vi "LVDimInterface.dic_release_service.vi"(0 "callBackID":i32, 5 "error in (no error)":errorcluster) -> (19 "error out":errorcluster)   [LabVIEW 2014, in "LVDimInterface.lvlib"]
doc: "Unregisters a control from a DIM service."
uses:
  LVDimInterface.lvlib
  bin/libDimWrapper.dll
  bin/libDimWrapper.so
  bin/libDimWrapperSPL.dll
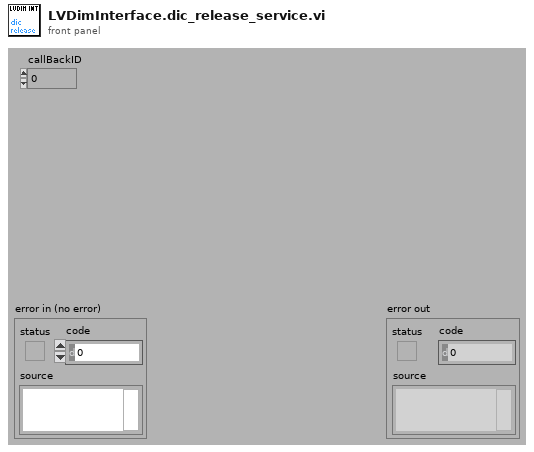
[diagram p1: front panel]
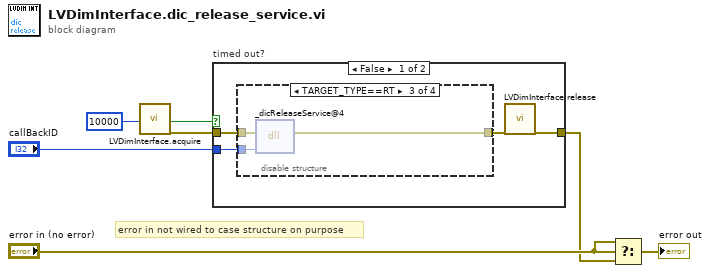
[diagram p0: block diagram]
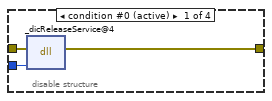
[diagram p2: hidden frame]
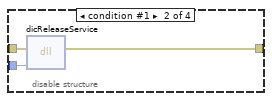
[diagram p3: hidden frame]
diagram:
  # "error in not wired to case structure on purpose"
  n1 = call "LVDimInterface.acquire.vi"("ms timeout (10000)"=10000 ("ms timeout (-1)")) -> ("timed out"=w5:bool, "error out"=w2:errorcluster)  [unwired: 17 in]
  n2 = case "timed out?" shown="False" w5 {
    tunnel: "callBackID" -> [w11 _]
    tunnel: w2 -> [w10 w22]
    tunnel: [w8 w22] -> w1
    frame False {
      n3 = disable-structure "Conditional Disable Structure" shown="TARGET_TYPE==RT" {
        disable-tunnel: w11 -> [w14 w17 w20 _]
        disable-tunnel: w10 -> [w13 w16 w19 w21]
        disable-tunnel: [w12 w15 w18 w21] -> w9
        frame condition #0 (active) {
          n4 = dll-call lib="D:/Git/CS-framework/CSlibraries-extern/DimLVEvent/bin/libDimWrapper.dll" fn="_dicReleaseService@4" label="dic_release_service"(error in=w13, "callBackID"=w14) -> (error out=w12:errorcluster)  [unwired: 4 in, 1 out]
        }
        frame condition #1 {
          n5 = dll-call lib="D:/Git/CS-framework/CSlibraries/DimLVEvent/bin/libDimWrapper.so" fn="dicReleaseService"(error in=w16, "callBackID"=w17) -> (error out=w15:errorcluster)  [unwired: 4 in, 1 out]
        }
        frame condition #2 {
          n6 = dll-call lib="D:/Git/CS-framework/CSlibraries/DimLVEvent/bin/libDimWrapperSPL.dll" fn="_dicReleaseService@4" label="libDimWrapper.so:dicReleaseService"(error in=w19, "callBackID"=w20) -> (error out=w18:errorcluster)  [unwired: 4 in, 1 out]
        }
        frame condition #3 {
        }
      }
      n7 = call "LVDimInterface.release.vi"("error in (no error)"=w9) -> ("error out"=w8:errorcluster)  [unwired: 18 in]
    }
    frame True {
    }
  }
  n8 = Select(t="error in (no error)", s="error in (no error)", f=w1) -> (s? t:f=→"error out":errorcluster)
